vi "Laser-On - 副本.vi"(2 "error in (no error)":errorcluster, 3 "SetLaserEnergy":dbl=10.0, 4 "standby":bool, 5 "VISA resource name":refnum<visa-resource-name>) -> (0 "error out":errorcluster, 1 "VISA resource name out":refnum<visa-resource-name>)   [LabVIEW 2013]
panel:
  # "uJ"
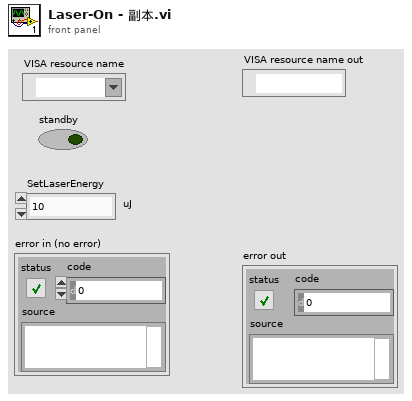
[diagram p1: front panel]
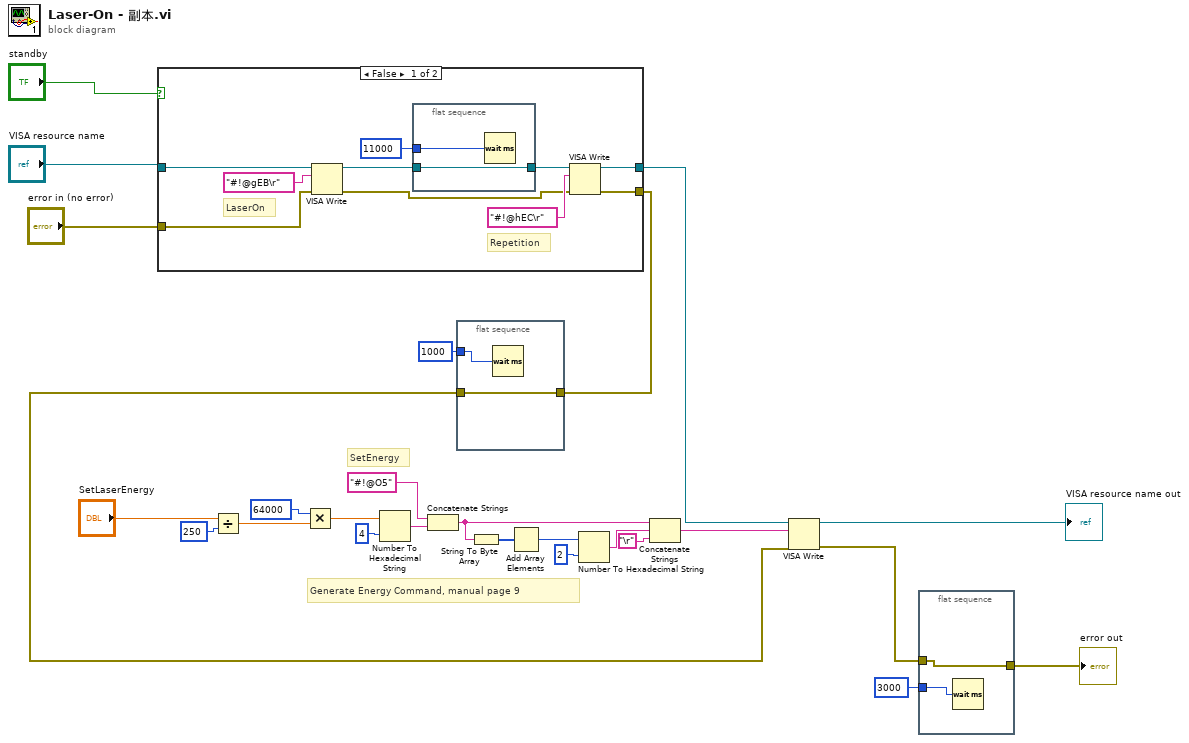
[diagram p0: block diagram]
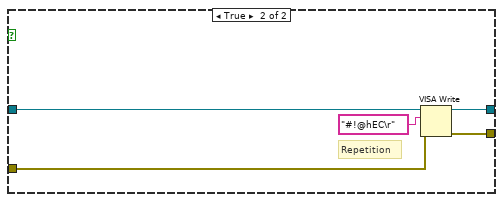
[diagram p2: hidden frame]
diagram:
  # "Generate Energy Command, manual page 9"
  # "SetEnergy"
  n1 = case shown="False" "standby" {
    tunnel: "VISA resource name" -> [w30 w42]
    tunnel: [w31 w41] -> w7
    tunnel: "error in (no error)" -> [w29 w40]
    tunnel: [w27 w39] -> w6
    frame False {
      # "LaserOn"
      # "Repetition"
      n2 = VISA Write(VISA resource name=w30, write buffer="#!@gEB\r", error in (no error)=w29) -> (VISA resource name out=w34:refnum<visa-resource-name>, error out=w28:errorcluster)  [unwired: 1 out]
      n3 = flat-sequence {
        tunnel: w34 -> [w38]
        tunnel: [w38] -> w32
        tunnel: u32 11000 ("delay before read (ms)") -> [w37]
        frame #0 {
          n4 = Wait (ms)(milliseconds to wait=w37) -> ()  [unwired: 1 out]
        }
      }
      n5 = VISA Write(VISA resource name=w32, write buffer="#!@hEC\r", error in (no error)=w28) -> (VISA resource name out=w31:refnum<visa-resource-name>, error out=w27:errorcluster)  [unwired: 1 out]
    }
    frame True {
      # "Repetition"
      n6 = VISA Write(VISA resource name=w42, write buffer="#!@hEC\r", error in (no error)=w40) -> (VISA resource name out=w41:refnum<visa-resource-name>, error out=w39:errorcluster)  [unwired: 1 out]
    }
  }
  n7 = Divide(x="SetLaserEnergy", y=250) -> (x/y=w13:dbl)
  n8 = Multiply(x=64000, y=w13) -> (x*y=w11:dbl)
  n9 = Number To Hexadecimal String(1:i16 4 ("width (-)"), 2:w11) -> (0:w22:string)
  n10 = Concatenate Strings("#!@O5" ("string"), w22) -> (w18:string)
  n11 = flat-sequence {
    tunnel: w6 -> [w45]
    tunnel: [w45] -> w5
    tunnel: 1000 -> [w44]
    frame #0 {
      n12 = Wait (ms)(milliseconds to wait=w44) -> ()  [unwired: 1 out]
    }
  }
  n13 = String To Byte Array(string=w18) -> (unsigned byte array=w21:u8[])
  n14 = Add Array Elements(numeric array=w21) -> (sum=w20:u8)
  n15 = Number To Hexadecimal String(1:i16 2 ("width (-)"), 2:w20) -> (0:w17:string)
  n16 = Concatenate Strings(w18, w17, "\r") -> (w9:string)
  n17 = VISA Write(VISA resource name=w7, write buffer=w9, error in (no error)=w5) -> (VISA resource name out=→"VISA resource name out":refnum<visa-resource-name>, error out=w3:errorcluster)  [unwired: 1 out]
  n18 = flat-sequence {
    tunnel: w3 -> [w47]
    tunnel: [w47] -> w2
    tunnel: 3000 -> [w46]
    frame #0 {
      n19 = Wait (ms)(milliseconds to wait=w46) -> ()  [unwired: 1 out]
    }
  }
  "error out" <- w2
